vi "List Units Panel 2.vi"(0 "System#":u8, 7 "Rack Number":i8=1 min=1 max=16 step=1, 8 "AutoAge.ini  File Path":path=path "\\\\Beco\\autoage/config/autoage.ini") -> ()   [LabVIEW 2021]
uses:
  Main Controls System v8.0/AutoAge Globals.vi
panel:
  in  "Update":bool=TRUE
  in  "Show Details":bool
  in  "40":bool
  in  "39":bool
  in  "38":bool
  in  "37":bool
  in  "36":bool
  in  "35":bool
  in  "34":bool
  in  "33":bool
  in  "32":bool
  in  "31":bool
  in  "30":bool
  in  "29":bool
  in  "28":bool
  in  "27":bool
  in  "26":bool
  in  "25":bool
  in  "24":bool
  in  "23":bool
  in  "22":bool
  in  "21":bool
  in  "20":bool
  in  "19":bool
  in  "18":bool
  in  "17":bool
  in  "16":bool
  in  "15":bool
  in  "14":bool
  in  "13":bool
  in  "12":bool
  in  "11":bool
  in  "10":bool
  in  "9":bool
  in  "8":bool
  in  "7":bool
  in  "6":bool
  in  "5":bool
  in  "4":bool
  in  "3":bool
  in  "2":bool
  in  "1":bool
  in  "Done":bool
  # "A red square in a position indicates that a  position is running."
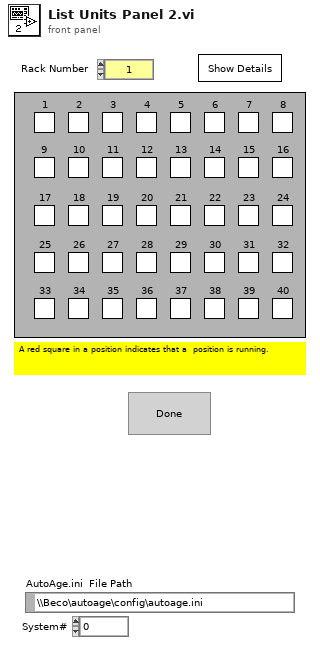
[diagram p1: front panel]
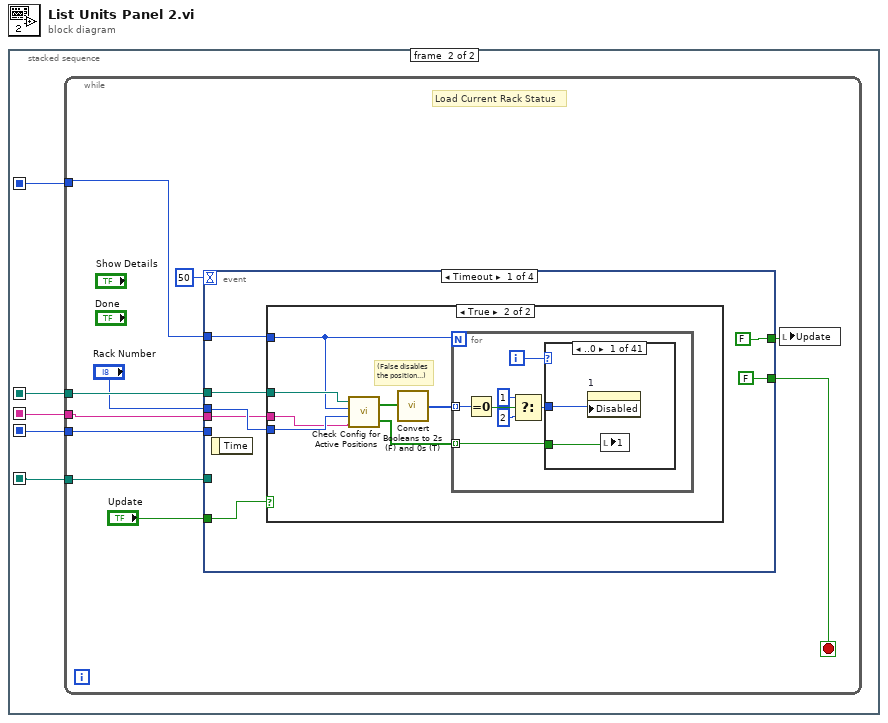
[diagram p0: block diagram]
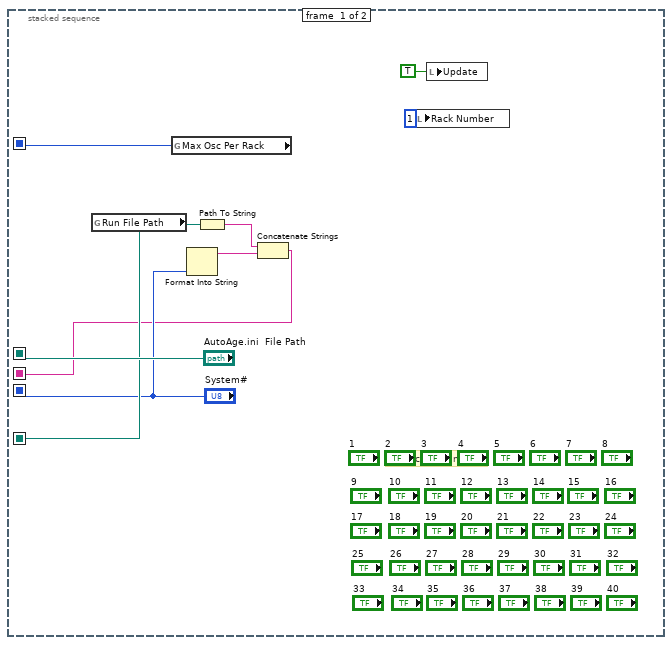
[diagram p2: hidden frame]
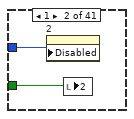
[diagram p4: hidden frame]
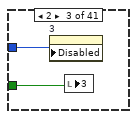
[diagram p5: hidden frame]
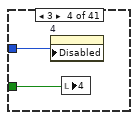
[diagram p6: hidden frame]
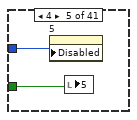
[diagram p7: hidden frame]
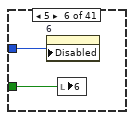
[diagram p8: hidden frame]
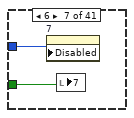
[diagram p9: hidden frame]
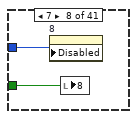
[diagram p10: hidden frame]
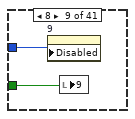
[diagram p11: hidden frame]
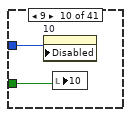
[diagram p12: hidden frame]
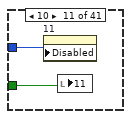
[diagram p13: hidden frame]
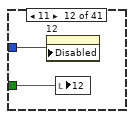
[diagram p14: hidden frame]
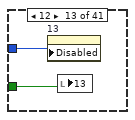
[diagram p15: hidden frame]
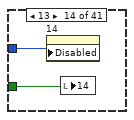
[diagram p16: hidden frame]
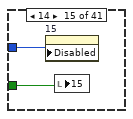
[diagram p17: hidden frame]
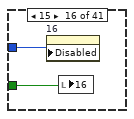
[diagram p18: hidden frame]
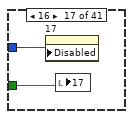
[diagram p19: hidden frame]
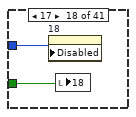
[diagram p20: hidden frame]
diagram:
  n1 = stacked-sequence {
    seq-local: ["AutoAge.ini  File Path" _] -> [_ w13]
    seq-local: [w3 _] -> [_ w12]
    seq-local: ["System#" _] -> [_ w11]
    seq-local: [w5 _] -> [_ w10]
    seq-local: [w2 _] -> [_ w14]
    frame #0 {
      # "The actual controls"
      n2 = global read "AutoAge Globals.vi" "Run File Path"() -> (w5:path)
      n3 = global read "AutoAge Globals.vi" "Max Osc Per Rack"() -> (w2:u16)
      n4 = Format Into String("System#") -> (resulting string=w7:string)  [unwired: 3 in, 1 out]
      n5 = Path To String(path=w5) -> (string=w8:string)
      n6 = Concatenate Strings(w8, w7) -> (w3:string)
      n7 = local write "Rack Number"(i8 1 ("Rack Number")) -> ()
      n8 = local write "Update"(TRUE ("Update")) -> ()
    }
    frame #1 {
      n9 = while {
        tunnel: w10 -> [w19]
        tunnel: w11 -> [w20]
        tunnel: w14 -> [w23]
        tunnel: w12 -> [w21]
        tunnel: w13 -> [w24]
        stop <- w18 stop-if-true
        # "Load Current Rack Status"
        n10 = event shown="[0] Timeout" {
          selector: _ -> [_ _ _ _]
          dyn-events: _ -> [_ _ _ _]
          timeout: 50 -> [_ _ _ _]
          tunnel: w20 -> [_ w133 _ _]
          tunnel: w19 -> [_ w132 _ _]
          tunnel: w23 -> [w28 _ _ _]
          tunnel: w24 -> [w29 w131 _ _]
          tunnel: [FALSE ("t") FALSE ("t") FALSE ("t") w144] -> w18
          tunnel: w21 -> [w25 _ _ _]
          tunnel: "Rack Number" -> [w30 w128 _ _]
          tunnel: [FALSE TRUE TRUE TRUE] -> w16
          tunnel: "Update" -> [w26 _ _ _]
          event Timeout {
            n11 = event-data() -> ()  [unwired: 1 in, 1 out]
            n12 = case shown="True" w26 {
              tunnel: w30 -> [_ w36]
              tunnel: w29 -> [_ w37]
              tunnel: w28 -> [_ w35]
              tunnel: w25 -> [_ w34]
              frame False {
              }
              frame True {
                # "(False disables\nthe position...)"
                n13 = call "Check Config for Active Positions.vi"("Run FilePath"=w34, "Rack Number"=w36, "Max Osc Per Rack"=w35, "AutoAge.ini  File Path"=w37) -> ("Active Positions"=w33:bool[], "Enabled Positions"=w32:bool[])
                n14 = call "Convert Booleans to 2s (F) and 0s (T)"("Boolean Array"=w32) -> ("2s and 0s"=w38:i8[])
                n15 = for {
                  N: w35 -> [_]
                  tunnel: w38 -> [w43] mode=indexing
                  tunnel: w33 -> [w45] mode=indexing
                  i -> [w44]
                  n16 = Equal To 0?(x=w43) -> (x = 0?=w41:bool)
                  n17 = Select(t=u8 1, s=w41, f=u8 2) -> (s? t:f=w42:u8)
                  n18 = case shown="..0" w44 {
                    tunnel: w42 -> [w47 w49 w50 w52 w55 w57 w59 w61 w63 w65 w67 w68 w71 w73 w75 w77 w79 w81 w83 w85 w87 w89 w91 w93 w95 w97 w99 w101 w103 w105 w107 w109 w111 w113 w115 w117 w119 w121 w123 w125 _]
                    tunnel: w45 -> [w46 w48 w51 w53 w54 w56 w58 w60 w62 w64 w66 w69 w70 w72 w74 w76 w78 w80 w82 w84 w86 w88 w90 w92 w94 w96 w98 w100 w102 w104 w106 w108 w110 w112 w114 w116 w118 w120 w122 w124 _]
                    frame ..0 {
                      n19 = property on="1" class="Bool (strict)"("Disabled"=w47) -> ()  [unwired: 2 in, 2 out]
                      n20 = local write "1"(w46) -> ()
                    }
                    frame 1 {
                      n21 = property on="2" class="Bool (strict)"("Disabled"=w49) -> ()  [unwired: 2 in, 2 out]
                      n22 = local write "2"(w48) -> ()
                    }
                    frame 2 {
                      n23 = property on="3" class="Bool (strict)"("Disabled"=w50) -> ()  [unwired: 2 in, 2 out]
                      n24 = local write "3"(w51) -> ()
                    }
                    frame 3 {
                      n25 = property on="4" class="Bool (strict)"("Disabled"=w52) -> ()  [unwired: 2 in, 2 out]
                      n26 = local write "4"(w53) -> ()
                    }
                    frame 4 {
                      n27 = property on="5" class="Bool (strict)"("Disabled"=w55) -> ()  [unwired: 2 in, 2 out]
                      n28 = local write "5"(w54) -> ()
                    }
                    frame 5 {
                      n29 = property on="6" class="Bool (strict)"("Disabled"=w57) -> ()  [unwired: 2 in, 2 out]
                      n30 = local write "6"(w56) -> ()
                    }
                    frame 6 {
                      n31 = property on="7" class="Bool (strict)"("Disabled"=w59) -> ()  [unwired: 2 in, 2 out]
                      n32 = local write "7"(w58) -> ()
                    }
                    frame 7 {
                      n33 = property on="8" class="Bool (strict)"("Disabled"=w61) -> ()  [unwired: 2 in, 2 out]
                      n34 = local write "8"(w60) -> ()
                    }
                    frame 8 {
                      n35 = property on="9" class="Bool (strict)"("Disabled"=w63) -> ()  [unwired: 2 in, 2 out]
                      n36 = local write "9"(w62) -> ()
                    }
                    frame 9 {
                      n37 = property on="10" class="Bool (strict)"("Disabled"=w65) -> ()  [unwired: 2 in, 2 out]
                      n38 = local write "10"(w64) -> ()
                    }
                    frame 10 {
                      n39 = property on="11" class="Bool (strict)"("Disabled"=w67) -> ()  [unwired: 2 in, 2 out]
                      n40 = local write "11"(w66) -> ()
                    }
                    frame 11 {
                      n41 = property on="12" class="Bool (strict)"("Disabled"=w68) -> ()  [unwired: 2 in, 2 out]
                      n42 = local write "12"(w69) -> ()
                    }
                    frame 12 {
                      n43 = property on="13" class="Bool (strict)"("Disabled"=w71) -> ()  [unwired: 2 in, 2 out]
                      n44 = local write "13"(w70) -> ()
                    }
                    frame 13 {
                      n45 = property on="14" class="Bool (strict)"("Disabled"=w73) -> ()  [unwired: 2 in, 2 out]
                      n46 = local write "14"(w72) -> ()
                    }
                    frame 14 {
                      n47 = property on="15" class="Bool (strict)"("Disabled"=w75) -> ()  [unwired: 2 in, 2 out]
                      n48 = local write "15"(w74) -> ()
                    }
                    frame 15 {
                      n49 = property on="16" class="Bool (strict)"("Disabled"=w77) -> ()  [unwired: 2 in, 2 out]
                      n50 = local write "16"(w76) -> ()
                    }
                    frame 16 {
                      n51 = property on="17" class="Bool (strict)"("Disabled"=w79) -> ()  [unwired: 2 in, 2 out]
                      n52 = local write "17"(w78) -> ()
                    }
                    frame 17 {
                      n53 = property on="18" class="Bool (strict)"("Disabled"=w81) -> ()  [unwired: 2 in, 2 out]
                      n54 = local write "18"(w80) -> ()
                    }
                    frame 18 {
                      n55 = property on="19" class="Bool (strict)"("Disabled"=w83) -> ()  [unwired: 2 in, 2 out]
                      n56 = local write "19"(w82) -> ()
                    }
                    frame 19 {
                      n57 = property on="20" class="Bool (strict)"("Disabled"=w85) -> ()  [unwired: 2 in, 2 out]
                      n58 = local write "20"(w84) -> ()
                    }
                    frame 20 {
                      n59 = property on="21" class="Bool (strict)"("Disabled"=w87) -> ()  [unwired: 2 in, 2 out]
                      n60 = local write "21"(w86) -> ()
                    }
                    frame 21 {
                      n61 = property on="22" class="Bool (strict)"("Disabled"=w89) -> ()  [unwired: 2 in, 2 out]
                      n62 = local write "22"(w88) -> ()
                    }
                    frame 22 {
                      n63 = property on="23" class="Bool (strict)"("Disabled"=w91) -> ()  [unwired: 2 in, 2 out]
                      n64 = local write "23"(w90) -> ()
                    }
                    frame 23 {
                      n65 = property on="24" class="Bool (strict)"("Disabled"=w93) -> ()  [unwired: 2 in, 2 out]
                      n66 = local write "24"(w92) -> ()
                    }
                    frame 24 {
                      n67 = property on="25" class="Bool (strict)"("Disabled"=w95) -> ()  [unwired: 2 in, 2 out]
                      n68 = local write "25"(w94) -> ()
                    }
                    frame 25 {
                      n69 = property on="26" class="Bool (strict)"("Disabled"=w97) -> ()  [unwired: 2 in, 2 out]
                      n70 = local write "26"(w96) -> ()
                    }
                    frame 26 {
                      n71 = property on="27" class="Bool (strict)"("Disabled"=w99) -> ()  [unwired: 2 in, 2 out]
                      n72 = local write "27"(w98) -> ()
                    }
                    frame 27 {
                      n73 = property on="28" class="Bool (strict)"("Disabled"=w101) -> ()  [unwired: 2 in, 2 out]
                      n74 = local write "28"(w100) -> ()
                    }
                    frame 28 {
                      n75 = property on="29" class="Bool (strict)"("Disabled"=w103) -> ()  [unwired: 2 in, 2 out]
                      n76 = local write "29"(w102) -> ()
                    }
                    frame 29 {
                      n77 = property on="30" class="Bool (strict)"("Disabled"=w105) -> ()  [unwired: 2 in, 2 out]
                      n78 = local write "30"(w104) -> ()
                    }
                    frame 30 {
                      n79 = property on="31" class="Bool (strict)"("Disabled"=w107) -> ()  [unwired: 2 in, 2 out]
                      n80 = local write "31"(w106) -> ()
                    }
                    frame 31 {
                      n81 = property on="32" class="Bool (strict)"("Disabled"=w109) -> ()  [unwired: 2 in, 2 out]
                      n82 = local write "32"(w108) -> ()
                    }
                    frame 32 {
                      n83 = property on="33" class="Bool (strict)"("Disabled"=w111) -> ()  [unwired: 2 in, 2 out]
                      n84 = local write "33"(w110) -> ()
                    }
                    frame 33 {
                      n85 = property on="34" class="Bool (strict)"("Disabled"=w113) -> ()  [unwired: 2 in, 2 out]
                      n86 = local write "34"(w112) -> ()
                    }
                    frame 34 {
                      n87 = property on="35" class="Bool (strict)"("Disabled"=w115) -> ()  [unwired: 2 in, 2 out]
                      n88 = local write "35"(w114) -> ()
                    }
                    frame 35 {
                      n89 = property on="36" class="Bool (strict)"("Disabled"=w117) -> ()  [unwired: 2 in, 2 out]
                      n90 = local write "36"(w116) -> ()
                    }
                    frame 36 {
                      n91 = property on="37" class="Bool (strict)"("Disabled"=w119) -> ()  [unwired: 2 in, 2 out]
                      n92 = local write "37"(w118) -> ()
                    }
                    frame 37 {
                      n93 = property on="38" class="Bool (strict)"("Disabled"=w121) -> ()  [unwired: 2 in, 2 out]
                      n94 = local write "38"(w120) -> ()
                    }
                    frame 38 {
                      n95 = property on="39" class="Bool (strict)"("Disabled"=w123) -> ()  [unwired: 2 in, 2 out]
                      n96 = local write "39"(w122) -> ()
                    }
                    frame 39 {
                      n97 = property on="40" class="Bool (strict)"("Disabled"=w125) -> ()  [unwired: 2 in, 2 out]
                      n98 = local write "40"(w124) -> ()
                    }
                    frame 40, Default {
                    }
                  }
                }
              }
            }
          }
          event "Show Details": Value Change {
            n99 = event-data() -> ("NewVal"=w129:bool)  [unwired: 1 in]
            n100 = case shown="True" w129 {
              tunnel: w133 -> [_ w139]
              tunnel: w132 -> [_ w137]
              tunnel: w131 -> [_ w138]
              tunnel: w128 -> [w134 w136]
              tunnel: [w134 w135] -> w126
              frame False {
              }
              frame True {
                n101 = call "Show Rack Details"("Sytem #"=w139, "AutoAge.ini File Path"=w138, "Pos.run File Path"=w137, "Rack"=w136) -> ("New Rack"=w135:i8)
              }
            }
            n102 = local write "Rack Number"(w126) -> ()
          }
          event "Rack Number": Value Change {
            # "Use local variables to preload the controls with the existing status of the position.\nUse an attribute node to disable the control for positions that are already running."
            n103 = event-data() -> ("NewVal"=w140:i8)  [unwired: 1 in]
            n104 = local write "Rack Number"(w140) -> ()
          }
          event "Done": Value Change {
            n105 = event-data() -> ("NewVal"=w144:bool)  [unwired: 1 in]
          }
        }
        n106 = local write "Update"(w16) -> ()
      }
    }
  }
